vi "Write Block Values.vi"(8 "error in (no error)":errorcluster, 9 "Write Block":u16[](array[numeric]) format="%04x", 10 "Start Index":i32, 11 "Virtual Memory Unit in":refnum<class "Virtual Memory Unit.lvclass">) -> (0 "error out":errorcluster, 3 "Virtual Memory Unit out":refnum<class "Virtual Memory Unit.lvclass">)   [LabVIEW 2020, in "BCI-1553 API.lvlib" / "Virtual Memory.lvlib" / "Virtual Memory Unit.lvclass"]
doc: "Write a contiguous block into memory."
uses:
  Virtual Memory Unit.lvclass
  Virtual Memory Unit.lvclass/Virtual Memory Unit.ctl
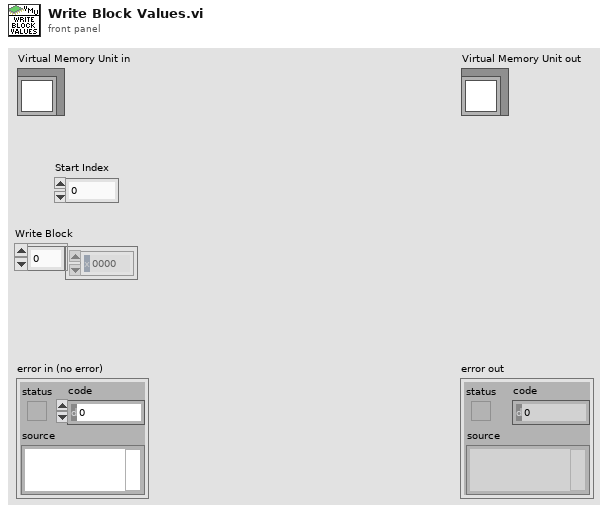
[diagram p1: front panel]
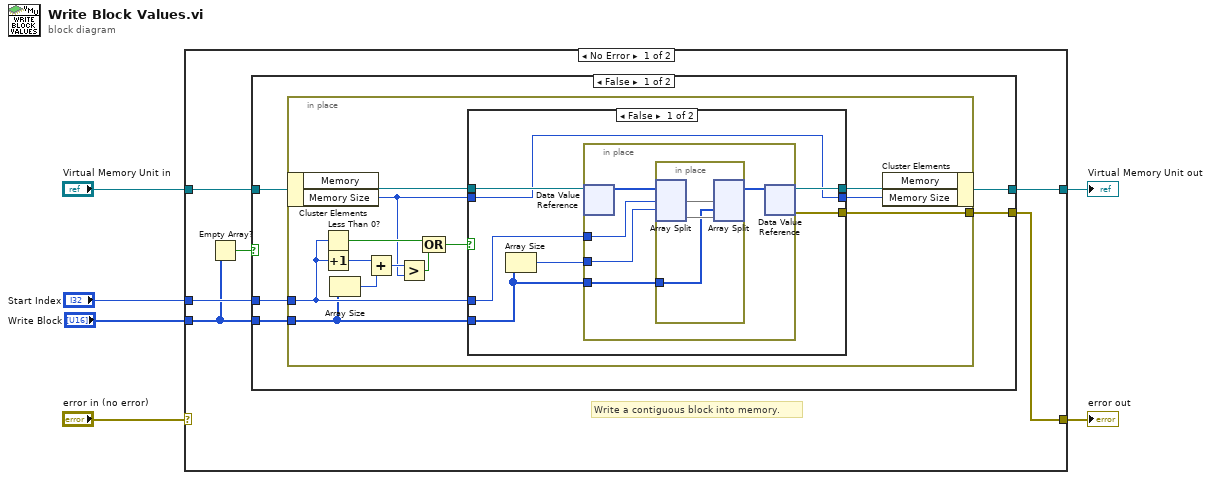
[diagram p0: block diagram]
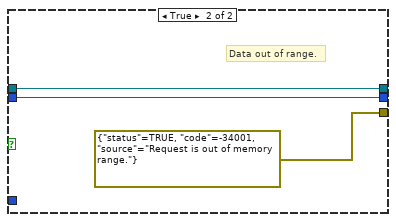
[diagram p2: hidden frame]
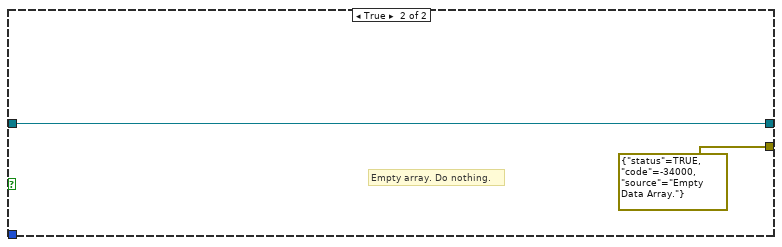
[diagram p3: hidden frame]
diagram:
  n1 = case shown="No Error" "error in (no error)" {
    selector: "error in (no error)" -> [_ w52]
    tunnel: [w7 w52] -> w5
    tunnel: [w11 w51] -> w3
    tunnel: "Virtual Memory Unit in" -> [w12 w51]
    tunnel: "Start Index" -> [w9 _]
    tunnel: "Write Block" -> [w8 _]
    frame No Error {
      # "Write a contiguous block into memory."
      n2 = Empty Array?(array=w8) -> (empty?=w10:bool)
      n3 = case shown="False" w10 {
        tunnel: w12 -> [w17 w50]
        tunnel: [w16 w50] -> w11
        tunnel: w9 -> [w15 _]
        tunnel: w8 -> [w14 _]
        tunnel: [w13 errorcluster {"status"=TRUE, "code"=-34000, "source"="Empty Data Array."} ("error IO")] -> w7
        frame False {
          n4 = in-place {
            in-place-border: w15 -> [w21]
            in-place-border: w14 -> [w20]
            in-place-border: [w28] -> w13
            n5 = in-place-cluster #1(w17) -> ("Memory"=w30:refnum<data-value>, "Memory Size"=w19:i32)
            n6 = Less Than 0?(x=w21) -> (x < 0?=w23:bool)
            n7 = Increment(x=w21) -> (x+1=w24:i32)
            n8 = Array Size(array=w20) -> (size(s)=w27:i32)
            n9 = Add(x=w24, y=w27) -> (x+y=w26:i32)
            n10 = Greater?(x=w26, y=w19) -> (0:w22:bool)
            n11 = Compound Arithmetic op=OR(w23, w22) -> (w25:bool)
            n12 = case shown="False" w25 {
              tunnel: w30 -> [w37 w48]
              tunnel: [w36 w48] -> w29
              tunnel: [w35 errorcluster {"status"=TRUE, "code"=-34001, "source"="Request is out of memory range."} ("error IO")] -> w28
              tunnel: w21 -> [w31 _]
              tunnel: w20 -> [w32 _]
              tunnel: w19 -> [w34 w47]
              tunnel: [w34 w47] -> w18
              frame False {
                n13 = Array Size(array=w32) -> (size(s)=w33:i32)
                n14 = in-place {
                  in-place-border: w31 -> [w40]
                  in-place-border: w33 -> [w39]
                  in-place-border: w32 -> [w38]
                  n15 = in-place-dvr #2(w37) -> (w42:u16[])  [unwired: 1 out]
                  n16 = in-place {
                    in-place-border: w38 -> [w43]
                    n17 = in-place-split #3(w42, w40, w39) -> (w45:u16[], w44:u16[])  [unwired: 1 out]
                    n18 = in-place-split #3(w45, w43, w44) -> (w41:u16[])  [unwired: 2 out]
                  }
                  n19 = in-place-dvr #2(w41) -> (w36:refnum<data-value>, w35:errorcluster)
                }
              }
              frame True {
                # "Data out of range."
              }
            }
            n20 = in-place-cluster #1("Memory"=w29, "Memory Size"=w18) -> (w16:refnum<class "Virtual Memory Unit.lvclass">)
          }
        }
        frame True {
          # "Empty array. Do nothing."
        }
      }
    }
    frame Error {
    }
  }
  "error out" <- w5
  "Virtual Memory Unit out" <- w3
